vi "PH_Cont-601k_PowerUnit.constructor.vi"(0 "name":string, 2 "data in":string, 5 "error in(no error)":errorcluster) -> (14 "i ref out":refnum<vi>, 16 "data out":string, 19 "error out":errorcluster)   [LabVIEW 2014, in "PH_Cont-601k_PowerUnit.lvlib"]
doc: "This class is forseen to control a PreAmp Power Unit. Actually it controls several device layer classes. The head itself is fully operational, but should be used via the PHELIX_Sequencer class only. It has an own state machine.\n\nThis class is part of the PHELIX application layer.\n\nauthor: Stefan Götte, GSI\n\nLicense Agreement for this software:\n\nCopyright (C)\nGesellschaft für Schwerionenforschung, GSI\nPlanckstr. 1\n64291 Darmstadt\nGermany\n\nContact: D.Beck@gsi.de \n\nThis program is free software; you can redistribute it and/or modify it under the terms of the \nGNU General Public License as published by the Free Software Foundation; either version 2 of \nthe license, or (at your option) any later version.\n\nThis program is distributed in the hope that it will be useful, but WITHOUT ANY WARRANTY; \nwithout even the implied warranty of MERCHANTABILITY or FITNESS FOR A PARTICULAR PURPOSE. See the GNU General License for more details (http://www.gnu.org).\n\nGesellschaft für Schwerionenforschung, GSI\nPlanckstr. 1, 64291 Darmstadt, Germany\nFor all questions and ideas contact: M.Richter@gsi.de, H.Brand@gsi.de or D.Beck@gsi.de.\nLast update: 16-JUN-2004"
uses:
  PH_Cont-601k_PowerUnit.lvlib
  PH_Basics/PH_PowerUnit_BaseClass/PH_PowerUnit_BaseClass.lvlib
  PH_Devices/PH_Cont-601k_PSU/PH_Cont-601k_PSU.lvlib
  PH_Basics/PH_Class/PH_Class.lvlib
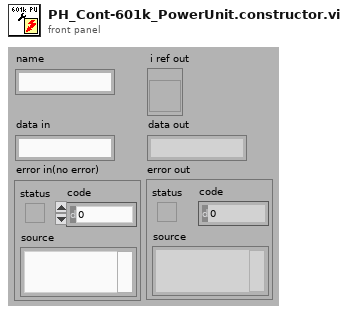
[diagram p1: front panel]
types:
  T1 = enum16{"SetAttribute", "GetAttribute", "CreateAttribute", "DestroyAttribute", "DestroyAllAtributes"}
  T2 = typedef "PH_Cont-601k_PowerUnit.lvlib/PH_Cont-601k_PowerUnit.i attribute.ctl" = cluster{"Service ID Last Shot":i32}
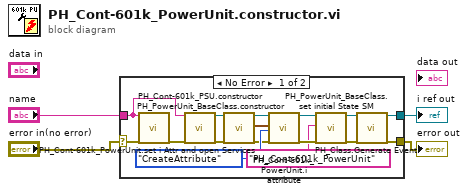
[diagram p0: block diagram]
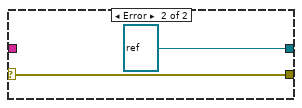
[diagram p2: hidden frame]
diagram:
  n1 = case shown="No Error" "error in(no error)" {
    selector: "error in(no error)" -> [w5 w22]
    tunnel: "name" -> [w6 _]
    tunnel: [w7 w22] -> w3
    tunnel: [w9 refnum<vi> refnum ("i ref out")] -> w2
    frame No Error {
      n2 = call "PH_PowerUnit_BaseClass.constructor.vi"("name"=w6, "error in(no error)"=w5) -> ("error out"=w14:errorcluster)  [unwired: 15 in, 2 out]
      n3 = call "PH_Cont-601k_PSU.constructor.vi"("name"=w6, "error in(no error)"=w14) -> ("i ref out"=w15:refnum<vi>, "error out"=w16:errorcluster)  [unwired: 15 in, 1 out]
      n4 = call "PH_Cont-601k_PowerUnit.set i Attr and open Services.vi"("i ref in"=w15, "error in"=w16) -> ("i ref out"=w17:refnum<vi>, "i Attribhutes"=w18:T2, "error out"=w19:errorcluster)  [unwired: 15 in]
      n5 = call "PH_Cont-601k_PowerUnit.i attribute.vi"("VI Refnum"=w17, "CLASS.i attribute"=w18, "Action"=T1."CreateAttribute", "error in (no error)"=w19) -> ("VI Refnum out"=w13:refnum<vi>, "error out"=w12:errorcluster)  [unwired: 13 in, 1 out]
      n6 = call "PH_Class.Generate Event.vi"("i ref in"=w13, "Class"="PH_Cont-601k_PowerUnit", "error in (no error)"=w12) -> ("i ref out"=w10:refnum<vi>, "error out"=w8:errorcluster)  [unwired: 15 in]
      n7 = call "PH_PowerUnit_BaseClass.set initial State SM.vi"("VI in"=w10, "error in (no error)"=w8) -> ("VI out"=w9:refnum<vi>, "error out"=w7:errorcluster)  [unwired: 16 in]
    }
    frame Error {
    }
  }
  "i ref out" <- w2
  "error out" <- w3
